vi "Beeper.vi"(8 "error in (no error)":errorcluster, 9 "Beep (F: No)":bool, 10 "Enable Beeper (T: On)":bool=TRUE, 11 "VISA resource name":refnum<visa-resource-name>) -> (0 "error out":errorcluster, 3 "VISA resource name out":refnum<visa-resource-name>)   [LabVIEW 2017, in "Keithley 3390.lvlib"]
doc: "Enables or disables the function generator's beeper. Can also be used to beep the beeper."
uses:
  Keithley 3390.lvlib
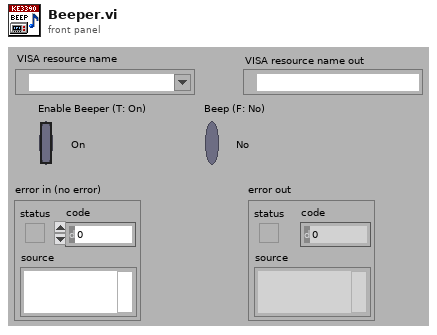
[diagram p1: front panel]
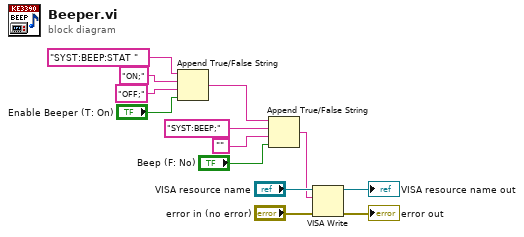
[diagram p0: block diagram]
diagram:
  n1 = Append True/False String(1:"Enable Beeper (T: On)", 2:"OFF;" ("false string"), 3:"ON;" ("true string"), 4:"SYST:BEEP:STAT " ("string (\"\")")) -> (0:w5:string)
  n2 = Append True/False String(1:"Beep (F: No)", 2:"", 3:"SYST:BEEP;" ("true string"), 4:w5) -> (0:w1:string)
  n3 = VISA Write(VISA resource name="VISA resource name", write buffer=w1, error in (no error)="error in (no error)") -> (VISA resource name out=→"VISA resource name out":refnum<visa-resource-name>, error out=→"error out":errorcluster)  [unwired: 1 out]
